vi "Test Worker Waiting After Completing Job.vi"(8 "error in (no error)":errorcluster, 11 "Cashier Test in":refnum<class "Cashier Test.lvclass">) -> (0 "error out":errorcluster, 3 "Cashier Test out":refnum<class "Cashier Test.lvclass">)   [LabVIEW 2020, in "Cashier Test.lvclass"]
uses:
  Cashier Test.lvclass
  C:/git/astemes-triarc-examples/source/Coffee Shop/Tests/Worker Test/Worker Test.lvclass
  C:/Program Files (x86)/National Instruments/LabVIEW 2020/vi.lib/Astemes/LUnit/Test Case.lvclass
  Support/Beverages/TypeDefs/Drink Type.ctl
  Support/Beverages/TypeDefs/Options.ctl
  Processes/People/Customers/Customer/Customer.lvclass
  Test Doubles/Stub Job Handler/Stub Job Handler.lvclass
  C:/git/astemes-triarc-examples/source/Coffee Shop/Processes/People/Process Job/Job Handler.lvclass
  <vilib>/Astemes/Triarc Framework/Process/Process.lvclass/Process.ctl
  <vilib>/Astemes/LUnit/Test Case.lvclass/Test Case.ctl
  <vilib>/Astemes/Triarc Framework/Process/Public/Lifecycle/Get Lifecycle State.vi
  <vilib>/Astemes/Triarc Framework/Broadcast Event Helpers/Execution timer.vi
  <vilib>/Astemes/Triarc Framework/Process/Private/SubVIs/Wait for finish.vi
  <vilib>/Astemes/Triarc Framework/Process/Private/SubVIs/Set Lifecycle State.vi
  <vilib>/Astemes/Triarc Framework/Process/Protected/Messaging/Send Message.vi
  <vilib>/Astemes/LUnit/Append Pass Result.vi
  <vilib>/Astemes/LUnit/Append Fail Result.vi
  <vilib>/Utility/error.llb/Clear Errors.vi
  <vilib>/Astemes/Triarc Framework/Process/Private/SubVIs/Handle Debug Data.vi
  <vilib>/Astemes/Triarc Framework/Logging/Log Debug.vi
  <vilib>/AdvancedString/1D String Array to Delimited String.vi
  <vilib>/Utility/High Resolution Relative Seconds.vi
  Processes/People/Workers/Worker/Worker.lvclass
  C:/Program Files (x86)/National Instruments/LabVIEW 2020/vi.lib/Astemes/Triarc Framework/Process/Process.lvclass
  <vilib>/Utility/error.llb/Error Cluster From Error Code.vi
  <vilib>/Astemes/Triarc Framework/Support/Dequeue Broadcast Message.vi
  <vilib>/Astemes/Triarc Framework/Process/Public/Read Name.vi
  <vilib>/Astemes/Triarc Framework/Callback/Callback.lvclass
  <vilib>/Astemes/Triarc Framework/Process/Process.lvclass
  Cashier Test.lvclass/Cashier Test.ctl
  Worker Test/Worker Test.lvclass
  <vilib>/Astemes/LUnit/Test Case.lvclass
  Support/Order/Order.lvclass
  Support/Beverages/Beverage/Beverage.lvclass
  <vilib>/Astemes/Triarc Framework/Support/Broadcast Event Dequeuers.lvlib
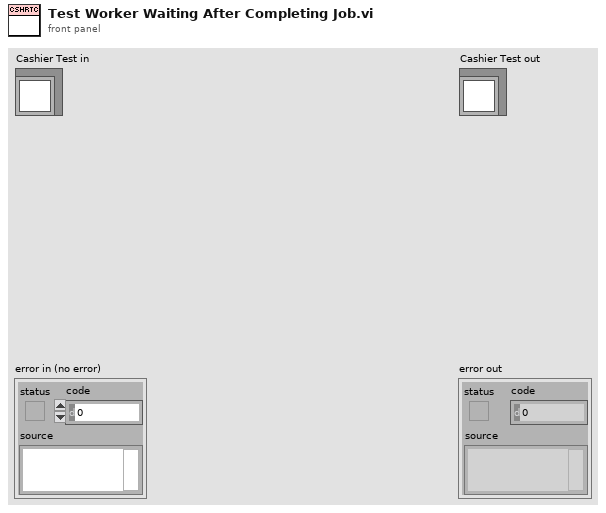
[diagram p1: front panel]
types:
  T1 = typedef "Beverage.lvclass/Drink Type.ctl" = enum16{"Dark Roast", "Decaf", "Espresso", "House Blend"}
  T2 = typedef "Beverage.lvclass/Options.ctl" = enum16{"<None>", "Milk", "Mocha", "Soy", "Whip"}
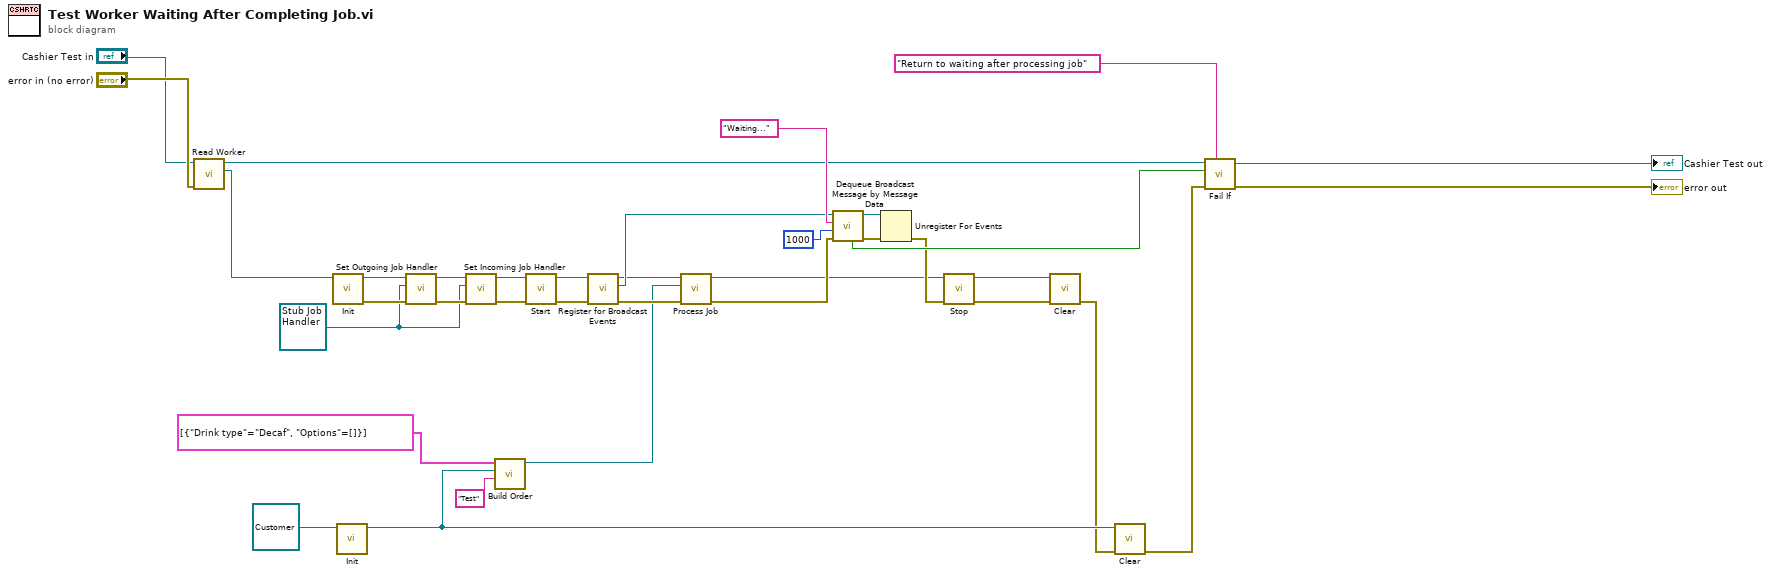
[diagram p0: block diagram]
diagram:
  w1 = refnum<class "Stub Job Handler.lvclass"> refnum ("Stub Job Processor.lvclass")
  n1 = call "Read Worker.vi"("error in (no error)"="error in (no error)", "Worker Test in"="Cashier Test in") -> ("Worker"=w15:refnum<class "Worker.lvclass">, "Worker Test out"=w14:refnum<class "Cashier Test.lvclass">)  [unwired: 7 in, 1 out]
  n2 = call-dynamic "Init.vi"("View In"=w15) -> ("error out"=w16:errorcluster, "View Out"=w6:refnum<class "Worker.lvclass">)  [unwired: 9 in]
  n3 = call-dynamic "Init.vi"("View In"=refnum<class "Customer.lvclass"> refnum ("Customer.lvclass")) -> ("View Out"=w10:refnum<class "Customer.lvclass">)  [unwired: 9 in, 1 out]
  n4 = call "Set Outgoing Job Handler.vi"("error in (no error)"=w16, "Work Dispatcher"=w1, "Worker In"=w6) -> ("error out"=w7:errorcluster, "Worker Out"=w4:refnum<class "Worker.lvclass">)  [unwired: 7 in]
  n5 = call "Set Incoming Job Handler.vi"("error in (no error)"=w7, "Job Handler"=w1, "Worker In"=w4) -> ("error out"=w5:errorcluster, "Worker Out"=w3:refnum<class "Worker.lvclass">)  [unwired: 7 in]
  n6 = call "Build Order.vi"("Customer Name"="Test", "Customer"=w10, "Order"=cluster{"Drink type":T1, "Options":T2[]}[] [{"Drink type"=enum."Decaf", "Options"=[]}]) -> ("Order Out"=w11:refnum<class "Order.lvclass">)  [unwired: 7 in, 1 out]
  n7 = call <vilib>:"Start.vi"("error in (no error)"=w5, "Process In"=w3) -> ("error out"=w19:errorcluster, "Process Out"=w22:refnum<class "Worker.lvclass">)  [unwired: 7 in, 1 out]
  n8 = call <vilib>:"Register for Broadcast Events.vi"("error in (no error)"=w19, "Process In"=w22) -> ("error out"=w21:errorcluster, "Event Registration Refnum Out"=w26:refnum<event-registration>, "Process Out"=w23:refnum<class "Worker.lvclass">)  [unwired: 7 in]
  n9 = call-dynamic "Process Job.vi"("error in (no error)"=w21, "Job"=w11, "Worker In"=w23) -> ("error out"=w25:errorcluster, "Worker Out"=w24:refnum<class "Worker.lvclass">)  [unwired: 7 in]
  n10 = call <vilib>:"Dequeue Broadcast Message by Message Data.vi"("error in (no error)"=w25, "Timeout (-1)"=1000, "Message Data"="Waiting...", "Event Registration Refnum"=w26) -> ("error out"=w29:errorcluster, "Event Registration Refnum Out"=w31:refnum<event-registration>, "Timed Out?"=w32:bool)  [unwired: 3 in, 2 out]
  n11 = Unregister For Events(event registration refnum=w31, error in=w29) -> (error out=w30:errorcluster)
  n12 = call <vilib>:"Stop.vi"("error in (no error)"=w30, "Process In"=w24) -> ("error out"=w18:errorcluster, "Process Out"=w17:refnum<class "Worker.lvclass">)  [unwired: 7 in, 1 out]
  n13 = call-dynamic "Clear.vi"("error in (no error)"=w18, "View In"=w17) -> ("error out"=w9:errorcluster)  [unwired: 9 in]
  n14 = call-dynamic "Clear.vi"("error in (no error)"=w9, "View In"=w10) -> ("error out"=w8:errorcluster)  [unwired: 9 in]
  n15 = call <vilib>:"Fail If.vi"("Description"="Return to waiting after processing job", "error in (no error)"=w8, "Fail?"=w32, "LUnit Test Case In"=w14) -> ("error out"=→"error out":errorcluster, "LUnit Test Case Out"=→"Cashier Test out":refnum<class "Cashier Test.lvclass">)  [unwired: 6 in]
